vi "output-save-spectra.vi"(0 "Wavelength Array":sgl[](array[numeric]), 1 "Raw Signal Array":i32[](array[numeric]), 2 "Background Array":i32[](array[numeric]), 3 "User Name":string, 4 "NAS Server ok?":bool, 5 "Save?":bool=TRUE, 6 "Header":string, 7 "Header for .ibw":string, 8 "File Name":string, 9 "Power (µW)":dbl format="%#_13g") -> ()   [LabVIEW 2017]
uses:
  Desktop/Programmierung PLE/user.lib (LabVIEW 32 bit)/IGOR Pro/igorBinV5.llb/single2D2ibw.vi
panel:
  in  "Indicator":i32
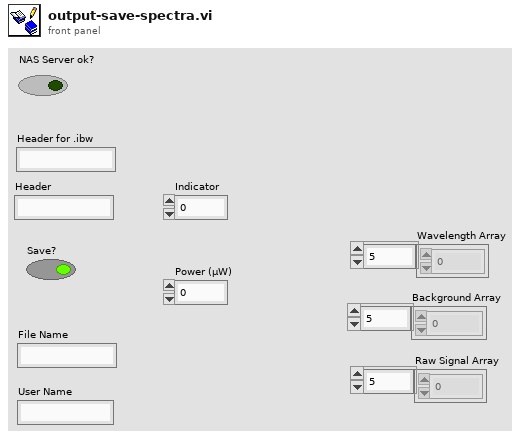
[diagram p1: front panel]
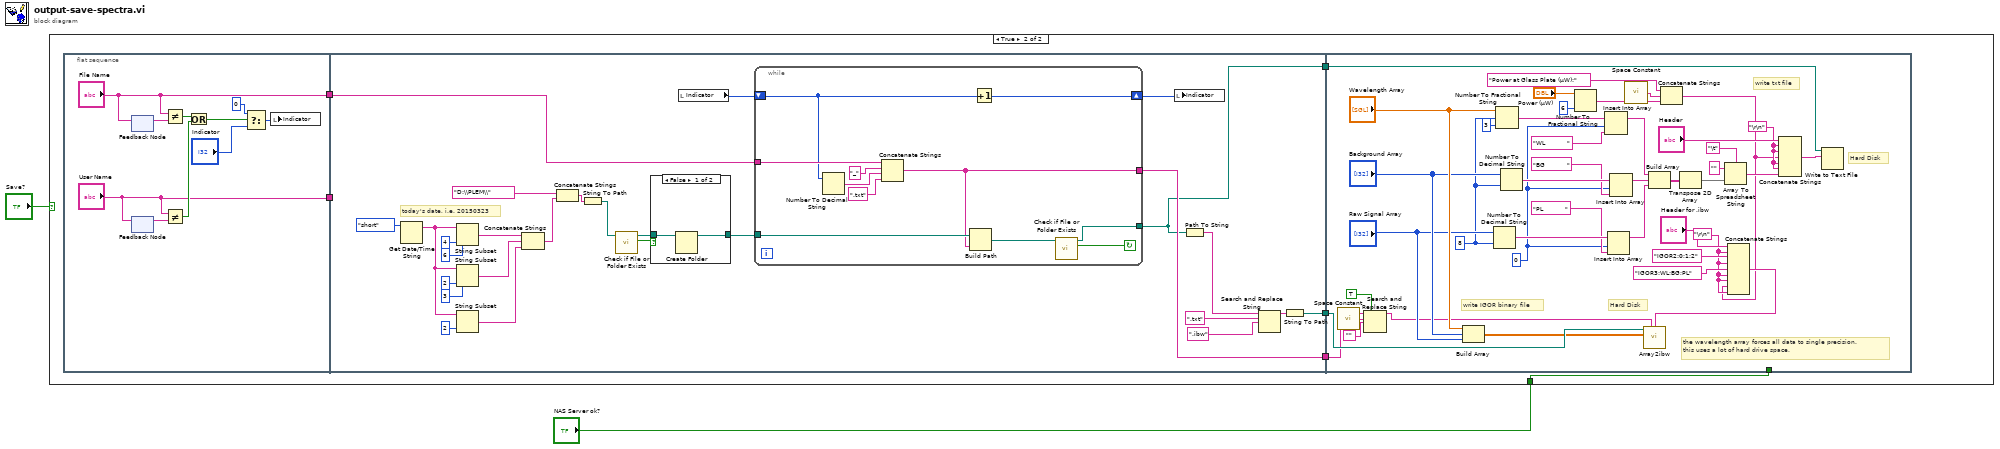
[diagram p0: block diagram]
diagram:
  n1 = case shown="True" "Save?" {
    tunnel: "NAS Server ok?" -> [_ w3]
    frame False {
    }
    frame True {
      n2 = flat-sequence {
        tunnel: ["File Name"] -> w8
        tunnel: ["User Name"] -> w5
        tunnel: w8 -> [w23]
        tunnel: [w30] -> w7
        tunnel: [w20] -> w6
        tunnel: w5 -> [_]
        tunnel: [w19] -> w4
        tunnel: w7 -> [w77]
        tunnel: w6 -> [w64]
        tunnel: w4 -> [w96]
        tunnel: w3 -> [_]
        frame #0 {
          n3 = feedback #1() -> (w10:string)  [unwired: 1 in]
          n4 = feedback-in #1("File Name") -> ()
          n5 = feedback #2() -> (w11:string)  [unwired: 1 in]
          n6 = feedback-in #2("User Name") -> ()
          n7 = Not Equal?(x="File Name", y=w10) -> (x != y?=w14:bool)
          n8 = Not Equal?(x="User Name", y=w11) -> (x != y?=w15:bool)
          n9 = Or(x=w14, y=w15) -> (x .or. y?=w13:bool)
          n10 = Select(t=0, s=w13, f="Indicator") -> (s? t:f=w16:i32)
          n11 = local write "Indicator"(w16) -> ()
        }
        frame #1 {
          # "today's date, i.e. 20150323"
          n12 = Get Date/Time String(date format (0)=enum16{"short", "long", "abbreviated"}."short") -> (date string=w45:string)  [unwired: 2 in, 1 out]
          n13 = String Subset(string=w45, offset (0)=6, length (rest)=4 ("length (rest)")) -> (substring=w42:string)
          n14 = String Subset(string=w45, offset (0)=3, length (rest)=2 ("length (rest)")) -> (substring=w43:string)
          n15 = String Subset(string=w45, length (rest)=2 ("length (rest)")) -> (substring=w44:string)  [unwired: 1 in]
          n16 = Concatenate Strings(w42, w43, w44) -> (w25:string)
          n17 = Concatenate Strings("D:\\PLEM\\" ("pszPath"), w25) -> (w35:string)
          n18 = String To Path(string=w35) -> (path=w32:path)
          n19 = call <vilib>:"Check if File or Folder Exists.vi"("path"=w32) -> ("file or folder exists?"=w33:bool, "dup path"=w34:path)  [unwired: 8 in, 1 out]
          n20 = case shown="False" w33 {
            tunnel: w34 -> [w58 w59]
            tunnel: [w57 w59] -> w24
            frame False {
              n21 = Create Folder(path (use dialog)=w58) -> (created path=w57:path)  [unwired: 2 in, 2 out]
            }
            frame True {
            }
          }
          n22 = local read "Indicator"() -> (w22:i32)
          n23 = while {
            tunnel: w24 -> [w56]
            tunnel: w23 -> [w54]
            shift-right: [w52] -> w21
            shift-left: w22 -> [w53]
            tunnel: [w48] -> w20
            tunnel: [w46] -> w19
            stop <- w55 continue-if-true
            n24 = Number To Decimal String(number=w53) -> (decimal integer string=w50:string)  [unwired: 1 in]
            n25 = Concatenate Strings(w54, "_" ("string"), w50, ".txt" ("string")) -> (w48:string)
            n26 = Build Path(base path=w56, name or relative path=w48) -> (appended path=w47:path)
            n27 = Increment(x=w53) -> (x+1=w52:i32)
            n28 = call <vilib>:"Check if File or Folder Exists.vi"("path"=w47) -> ("file or folder exists?"=w55:bool, "dup path"=w46:path)  [unwired: 8 in, 1 out]
          }
          n29 = local write "Indicator"(w21) -> ()
          n30 = Path To String(path=w19) -> (string=w29:string)
          n31 = Search and Replace String(input string=w29, search string=".txt", replace string=".ibw" ("replace string (\"\")")) -> (result string=w31:string)  [unwired: 5 in, 3 out]
          n32 = String To Path(string=w31) -> (path=w30:path)
        }
        frame #2 {
          w66 = "\r\n"
          w83 = 0 ("index")
          w74 = i16 8 ("width (-)")
          w72 = "\r\n"
          # "the wavelength array forces all data to single precision.\nthis uses a lot of hard drive space."
          # "Hard Disk"
          # "Hard Disk"
          # "write txt file"
          # "write IGOR binary file"
          n33 = call <vilib>:"Space Constant.vi"() -> ("String"=w62:string)
          n34 = Search and Replace String(replace all?=TRUE ("replace all? (F)"), input string=w64, search string=w62, replace string="") -> (result string=w60:string)  [unwired: 4 in, 3 out]
          n35 = Build Array("Wavelength Array", "Background Array", "Raw Signal Array") -> (w75:sgl[][])
          n36 = Number To Decimal String(number="Raw Signal Array", width (-)=w74) -> (decimal integer string=w90:string[])
          n37 = Number To Fractional String(number="Wavelength Array", width (-)=w74, precision (6)=i16 3) -> (F-format string=w91:string[])  [unwired: 1 in]
          n38 = Number To Decimal String(number="Background Array", width (-)=w74) -> (decimal integer string=w92:string[])
          n39 = Number To Fractional String(number="Power (µW)", precision (6)=i16 6) -> (F-format string=w71:string)  [unwired: 2 in]
          n40 = Insert Into Array(array=w91, index=w83, new element="WL           ") -> (w87:string[])
          n41 = Insert Into Array(array=w90, index=w83, new element="PL           ") -> (w88:string[])
          n42 = Insert Into Array(array=w92, index=w83, new element="BG           ") -> (w89:string[])
          n43 = call <vilib>:"Space Constant.vi"() -> ("String"=w70:string)
          n44 = Build Array(w87, w89, w88) -> (w97:string[][])
          n45 = Concatenate Strings("Power at Glass Plate (µW):", w70, w71) -> (w65:string)
          n46 = Transpose 2D Array(2D array=w97) -> (transposed array=w101:string[][])
          n47 = Array To Spreadsheet String(delimiter (Tab)="\t", array=w101, 3:"" ("format string")) -> (spreadsheet string=w73:string)
          n48 = Concatenate Strings("Header for .ibw", w66, "IGOR2:0;1;2", w66, "IGOR3:WL;BG;PL", w66, w66, w65, w66) -> (w76:string)
          n49 = call-poly "Array2ibw.vi"("path (default: dialog)"=w77, "wave name (\"wave0\")"=w60, "wave note (\"\")"=w76, "array in"=w75) -> ()  [unwired: 11 in, 1 out]
          n50 = Concatenate Strings("Header", w72, w72, w65, w72, w72, w73) -> (w78:string)
          n51 = Write to Text File(file (use dialog)=w96, text=w78) -> ()  [unwired: 2 in, 3 out]
        }
      }
    }
  }
